vi "gsp_simulator_global.vi"() -> ()   [LabVIEW 2015]
panel:
  in  "Port":refnum<visa-resource-name>
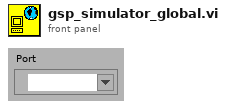
[diagram p1: front panel]
diagram:
